vi "Get Images and Freq.vi"(11 "Image Information Out":T1) -> (2 "upper limit":dbl, 3 "Array":string[](array[string]))   [LabVIEW 2013]
uses:
  ImageInfoList.ctl
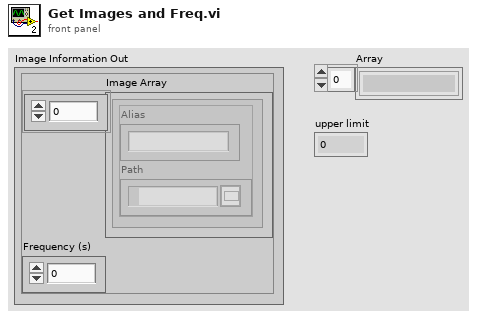
[diagram p1: front panel]
types:
  T1 = typedef "ImageInfoList.ctl" = cluster{"Image Array":cluster{"Alias":string, "Path":path}[], "Frequency (s)":dbl}
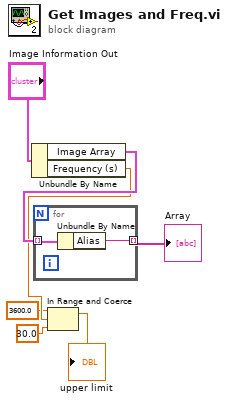
[diagram p0: block diagram]
diagram:
  n1 = Unbundle By Name("Image Information Out") -> ("Image Array"=w5:cluster{"Alias":string, "Path":path}[], "Frequency (s)"=w4:dbl)
  n2 = for {
    tunnel: w5 -> [w9] mode=indexing
    tunnel: [w8] -> w6 mode=indexing
    n3 = Unbundle By Name(w9) -> ("Alias"=w8:string)
  }
  "Array" <- w6
  n4 = In Range and Coerce(upper limit=3600.0, x=w4, lower limit=30.0) -> (coerced(x)=→"upper limit":dbl)  [unwired: 1 out]
